vi "BroadcastData.vi"(8 "error in (no error)":errorcluster, 10 "DataExchange":T1, 11 "GRMActor in":refnum<class "GenericController.lvclass">) -> (0 "error out":errorcluster, 3 "GRMActor out":refnum<class "GenericController.lvclass">)   [LabVIEW 2020, in "GenericController.lvlib" / "GenericController.lvclass"]
uses:
  GenericController.lvclass
  Device/Device/DataExchange.ctl
  GenericController.lvclass/GenericController.ctl
  Interface/DataListener Messages/OnDataChange Msg/OnDataChange Msg.lvclass/OnDataChange Msg.ctl
  <vilib>/ActorFramework/Message Enqueuer/Message Enqueuer.lvclass/Message Enqueuer.ctl
  <vilib>/ActorFramework/Message Enqueuer/Enqueue.vi
  Interface/DataListener Messages/OnDataChange Msg/OnDataChange Msg.lvclass
  C:/Program Files/National Instruments/LabVIEW 2020/vi.lib/ActorFramework/Message/Message.lvclass
  <vilib>/ActorFramework/Message Priority Queue/Priority Enqueue.vi
  Interface/DataListener/DataListener.lvclass
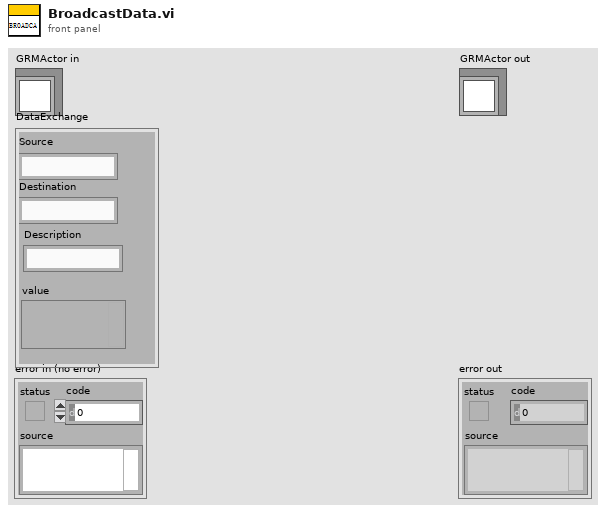
[diagram p1: front panel]
types:
  T1 = typedef "DataListener.lvclass/DataExchange.ctl" = cluster{"Source":string, "Destination":string, "Description":string, "value":variant}
  T2 = map{string, refnum<class "Message Enqueuer.lvclass">}
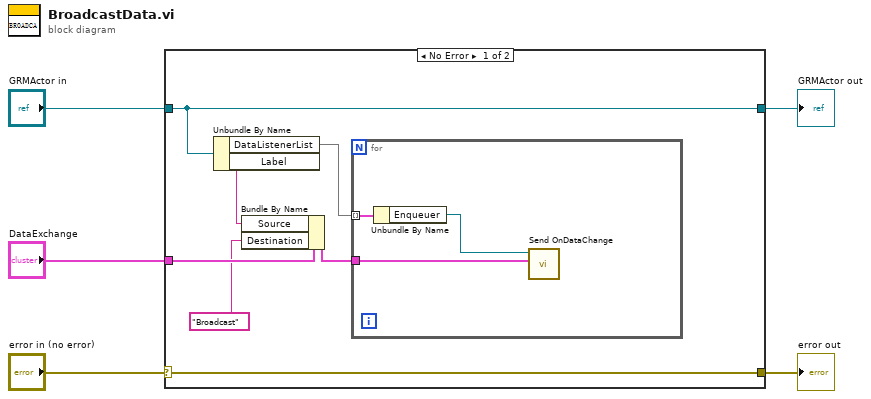
[diagram p0: block diagram]
diagram:
  n1 = case shown="No Error" "error in (no error)" {
    selector: "error in (no error)" -> [w12 w17]
    tunnel: [w12 w17] -> w2
    tunnel: [w11 w16] -> w1
    tunnel: "GRMActor in" -> [w11 w16]
    tunnel: "DataExchange" -> [w9 _]
    frame No Error {
      n2 = Unbundle By Name(w11) -> ("DataListenerList"=w10:T2, "Label"=w7:string)
      n3 = Bundle By Name(cluster=w9, "Source"=w7, "Destination"="Broadcast") -> (w8:T1)
      n4 = for {
        tunnel: w10 -> [w15] mode=indexing
        tunnel: w8 -> [w13]
        n5 = Unbundle By Name(w15) -> ("Enqueuer"=w14:refnum<class "Message Enqueuer.lvclass">)
        n6 = call "Send OnDataChange.vi"("DataExchange"=w13, "Message Enqueuer"=w14) -> ()  [unwired: 8 in, 2 out]
      }
    }
    frame Error {
    }
  }
  "error out" <- w2
  "GRMActor out" <- w1
